vi "Get InternalTemp.vi"(8 "error in (no error)":errorcluster, 11 "VISA resource name":refnum<visa-resource-name>) -> (0 "error out":errorcluster, 1 "InternalTemp (out)":dbl, 3 "VISA resource name out":refnum<visa-resource-name>)   [LabVIEW 2015, in "JULABO DeviceDriver.lvlib"]
doc: "This VI returns the actual temperature value measured by the internal bath sensor."
uses:
  JULABO DeviceDriver.lvlib
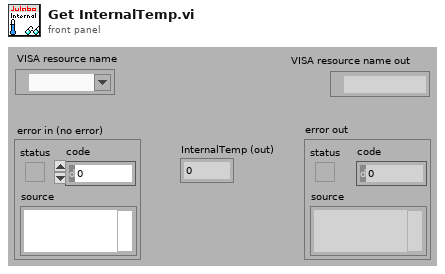
[diagram p1: front panel]
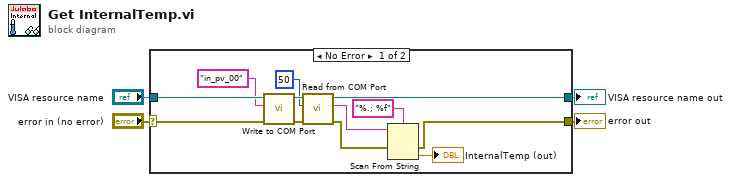
[diagram p0: block diagram]
diagram:
  n1 = case shown="No Error" "error in (no error)" {
    selector: "error in (no error)" -> [w15 w17]
    tunnel: "VISA resource name" -> [w16 w18]
    tunnel: [w8 w17] -> w2
    tunnel: [w7 w18] -> w1
    frame No Error {
      n2 = call "Write to COM Port.vi"("error in"=w15, "Command (input)"="in_pv_00", "VISA resource name in"=w16) -> ("error out"=w14:errorcluster, "VISA resource name out"=w13:refnum<visa-resource-name>)  [unwired: 7 in]
      n3 = call "Read from COM Port.vi"("error in"=w14, "Byte to Read (-1:All)"=u32 50 ("Anzahl der Byte"), "VISA resource name in"=w13) -> ("error out"=w11:errorcluster, "String (output)"=w10:string, "VISA resource name out"=w7:refnum<visa-resource-name>)  [unwired: 5 in, 1 out]
      n4 = Scan From String(format string="%.; %f" ("Format-String"), input string=w10, error in=w11) -> (error out=w8:errorcluster, output 1=→"InternalTemp (out)":dbl)  [unwired: 2 in, 2 out]
    }
    frame Error {
    }
  }
  "error out" <- w2
  "VISA resource name out" <- w1
